vi "public_device_occupy_choose_step.vi"(8 "error In":errorcluster, 9 "JSON string":string, 10 "Step order":string, 11 "process_ID":string) -> (0 "error IO":errorcluster)   [LabVIEW 2020]
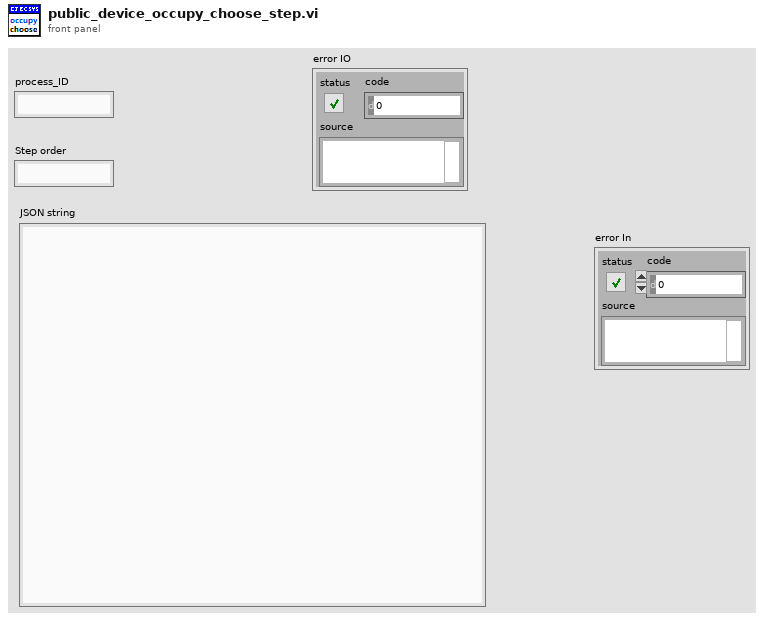
[diagram p1: front panel]
types:
  T1 = cluster{"status":bool, "code":i32, "string":string}
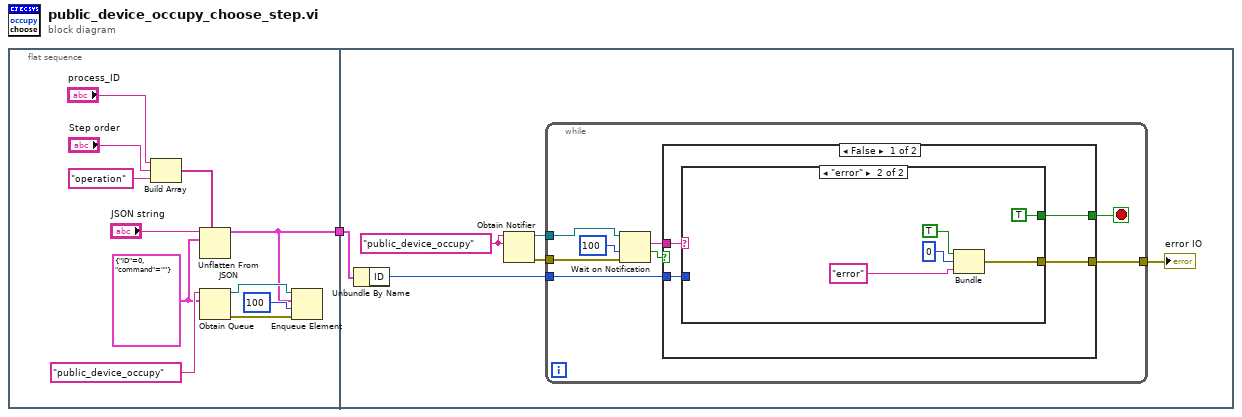
[diagram p0: block diagram]
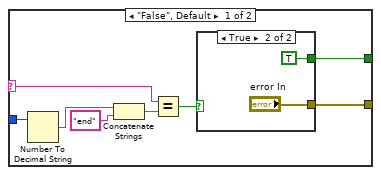
[diagram p2: hidden frame]
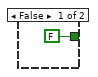
[diagram p3: hidden frame]
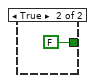
[diagram p4: hidden frame]
diagram:
  n1 = flat-sequence {
    tunnel: [w4] -> w1
    tunnel: w1 -> [w14]
    frame #0 {
      w2 = cluster{"ID":i32, "command":string} {"ID"=0, "command"=""} ("参数")
      n2 = Build Array("process_ID", "Step order", "operation" ("string")) -> (w10:string[])
      n3 = Unflatten From JSON(path=w10, JSON string="JSON string", type and defaults=w2) -> (value=w4:cluster{"ID":i32, "command":string})  [unwired: 4 in, 1 out]
      n4 = Obtain Queue(name (unnamed)="public_device_occupy", element data type=w2) -> (queue out=w11:refnum<queue>, error out=w12:errorcluster)  [unwired: 3 in, 1 out]
      n5 = Enqueue Element(queue=w11, element=w4, timeout in ms (-1)=100, error in (no error)=w12) -> ()  [unwired: 3 out]
    }
    frame #1 {
      w16 = "public_device_occupy" ("name (unnamed)")
      n6 = Unbundle By Name(w14) -> ("ID"=w13:i32)
      n7 = Obtain Notifier(name (unnamed)=w16, notification data type=w16) -> (notifier out=w18:refnum<notifier>, error out=w17:errorcluster)  [unwired: 2 in, 1 out]
      n8 = while {
        tunnel: w18 -> [w26]
        tunnel: w17 -> [w23]
        tunnel: [w20] -> w15
        tunnel: w13 -> [w19]
        stop <- w22 stop-if-true
        n9 = Wait on Notification(notifier=w26, timeout in ms (-1)=100, error in (no error)=w23) -> (notification=w21:string, timed out?=w24:bool)  [unwired: 1 in, 2 out]
        n10 = case shown="False" w24 {
          tunnel: [w29 FALSE] -> w22
          tunnel: w21 -> [w30 _]
          tunnel: [w28 _] -> w20
          tunnel: w19 -> [w27 _]
          frame False {
            n11 = case shown="\"error\"" w30 {
              selector: w30 -> [w38 _]
              tunnel: [w36 TRUE] -> w29
              tunnel: [w33 w43] -> w28
              tunnel: w27 -> [w32 _]
              frame "False", Default {
                n12 = Number To Decimal String(number=w32) -> (decimal integer string=w31:string)  [unwired: 1 in]
                n13 = Concatenate Strings(w31, "end" ("string")) -> (w34:string)
                n14 = Equal?(x=w38, y=w34) -> (x = y?=w37:bool)
                n15 = case shown="True" w37 {
                  tunnel: [FALSE TRUE] -> w36
                  tunnel: [_ "error In"] -> w33
                  frame False {
                  }
                  frame True {
                  }
                }
              }
              frame "error" {
                n16 = Bundle("status"=TRUE, "code"=0, "string"="error") -> (w43:T1)  [unwired: 1 in]
              }
            }
          }
          frame True {
          }
        }
      }
      "error IO" <- w15
    }
  }
